vi "Initialize.vi"(8 "error in (no error)":errorcluster, 11 "NI Galvo in":refnum<class "NI Galvo.lvclass">) -> (0 "error out":errorcluster, 3 "NI Galvo out":refnum<class "NI Galvo.lvclass">)   [LabVIEW 2014, in "NI Galvo.lvclass"]
uses:
  NI Galvo.lvclass
  NI Galvo.lvclass/NI Galvo.ctl
  <vilib>/DAQmx/create/channels.llb/DAQmx Create Channel (AO-Voltage-Basic).vi
  <vilib>/DAQmx/configure/timing.llb/DAQmx Timing (Sample Clock).vi
  <vilib>/DAQmx/write.llb/DAQmx Write (Analog 2D DBL NChan NSamp).vi
  Galvo.lvclass
  <resource>/objmgr/daqmx.rc
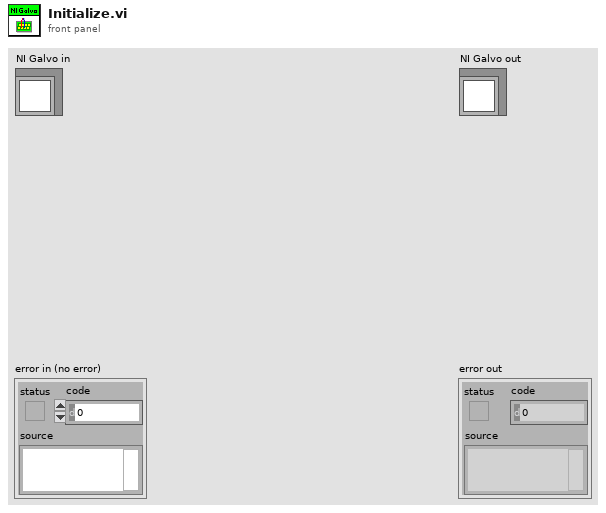
[diagram p1: front panel]
types:
  T1 = typedef "DAQ Class.lvclass/DAQ Parameters.ctl" = cluster{"Points Per A-Scan":u32, "A-Scans Per B-Scan":u32, "Number of B-Scans":u32, "A-Scans Per Transfer":u32, "Trigger Voltage":sgl, "Trigger Source":T2, "Trigger Slope":T3, "Channel":T4, "Clock":T5, "Bits per Sample":dbl, "Range":dbl}
  T2 = typedef "DAQ Class.lvclass/Trigger Source.ctl" = enum16{"External", "Channel A", "Channel B"}
  T3 = typedef "DAQ Class.lvclass/Trigger Slope.ctl" = enum16{"Rising", "Falling"}
  T4 = typedef "OCT DAQ Channel Data Type.ctl" = enum16{"Channel 1", "Channel 2", "Channel 1 and 2"}
  T5 = typedef "DAQ Class.lvclass/Clock Control.ctl" = enum16{"Internal Clock", "External Clock"}
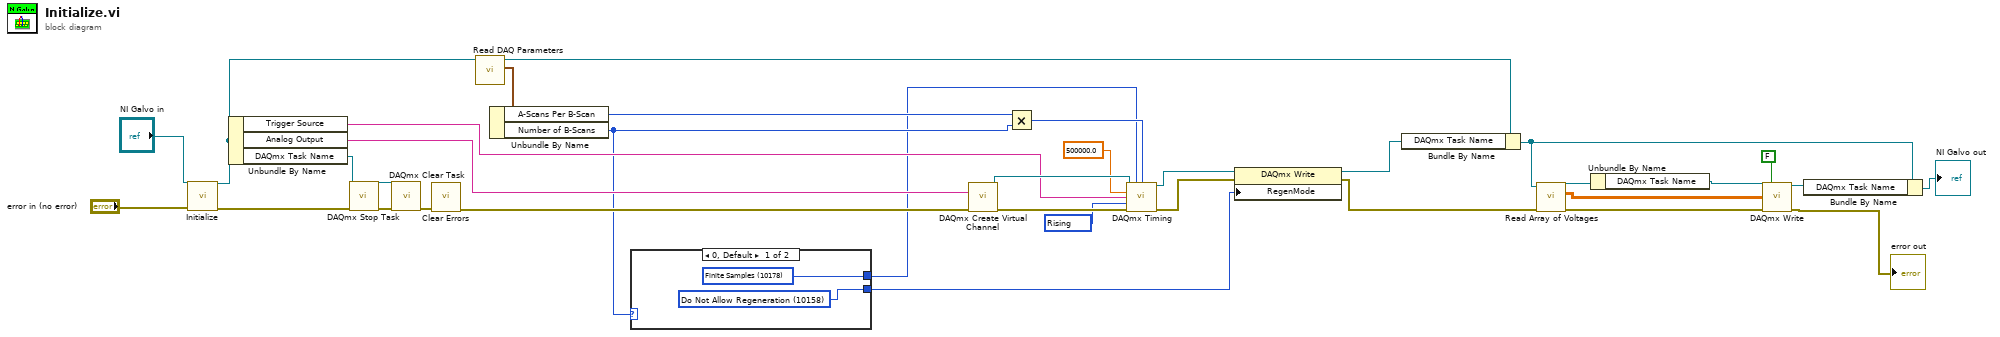
[diagram p0: block diagram]
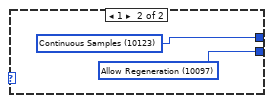
[diagram p2: hidden frame]
diagram:
  w27 = 10280 items=["Rising"=10280, "Falling"=10171] ("active edge")
  n1 = call-parent "Initialize.vi"("error in (no error)"="error in (no error)", "Galvo in"="NI Galvo in") -> ("error out"=w15:errorcluster, "Galvo out"=w17:refnum<class "NI Galvo.lvclass">)  [unwired: 8 in]
  n2 = Unbundle By Name(w17) -> ("Trigger Source"=w31:tag, "Analog Output"=w33:tag, "DAQmx Task Name"=w16:refnum<k21>)
  n3 = call <vilib>:"DAQmx Stop Task.vi"("task/channels in"=w16, "error in"=w15) -> ("task out"=w14:refnum<k21>, "error out"=w13:errorcluster)  [unwired: 12 in]
  n4 = call <vilib>:"DAQmx Clear Task.vi"("task in"=w14, "error in"=w13) -> ("error out"=w12:errorcluster)  [unwired: 13 in]
  n5 = call <vilib>:"Clear Errors.vi"("error in (no error)"=w12) -> ("error out"=w11:errorcluster)  [unwired: 5 in, 1 out]
  n6 = call-dynamic "Read DAQ Parameters.vi"("Galvo in"=w17) -> ("DAQ Parameters"=w19:T1, "Galvo out"=w20:refnum<class "NI Galvo.lvclass">)  [unwired: 8 in, 1 out]
  n7 = Unbundle By Name(w19) -> ("A-Scans Per B-Scan"=w18:u32, "Number of B-Scans"=w10:u32)
  n8 = case shown="0, Default" w10 {
    tunnel: [w37 w39] -> w1
    tunnel: [w36 w38] -> w8
    frame 0, Default {
      w36 = 10178 items=["Finite Samples"=10178, "Continuous Samples"=10123, "Hardware Timed Single Point"=12522] ("sample mode")
      w37 = 10158 items=["Allow Regeneration"=10097, "Do Not Allow Regeneration"=10158] ("RegenMode")
    }
    frame 1 {
      w38 = 10123 items=["Finite Samples"=10178, "Continuous Samples"=10123, "Hardware Timed Single Point"=12522] ("sample mode")
      w39 = 10097 items=["Allow Regeneration"=10097, "Do Not Allow Regeneration"=10158] ("RegenMode")
    }
  }
  n9 = call-poly <vilib>:"DAQmx Create Virtual Channel.vi"("physical channels"=w33, "error in"=w11) -> ("task out"=w32:refnum<k21>, "error out"=w30:errorcluster)  [unwired: 12 in]
  n10 = Multiply(x=w18, y=w10) -> (x*y=w28:u32)
  n11 = call-poly <vilib>:"DAQmx Timing.vi"("task/channels in"=w32, "sample mode"=w8, "samples per channel"=w28, "rate"=500000.0, "source"=w31, "active edge"=w27, "error in"=w30) -> ("task out"=w3:refnum<k21>, "error out"=w2:errorcluster)  [unwired: 7 in]
  n12 = property class="DAQmx Write"(reference=w3, error in=w2, "RegenMode"=w1) -> (reference out=w6:refnum<k21>, error out=w5:errorcluster)
  n13 = Bundle By Name(cluster=w20, "DAQmx Task Name"=w6) -> (w21:refnum<class "NI Galvo.lvclass">)
  n14 = call-dynamic "Read Array of Voltages.vi"("error in (no error)"=w5, "Galvo in"=w21) -> ("error out"=w22:errorcluster, "Array of Voltages"=w23:dbl[][], "Galvo out"=w25:refnum<class "NI Galvo.lvclass">)  [unwired: 7 in]
  n15 = Unbundle By Name(w25) -> ("DAQmx Task Name"=w24:refnum<k21>)
  n16 = call-poly <vilib>:"DAQmx Write.vi"("task/channels in"=w24, "auto start"=FALSE, "data"=w23, "error in"=w22) -> ("task out"=w7:refnum<k21>, "error out"=→"error out":errorcluster)  [unwired: 9 in, 1 out]
  n17 = Bundle By Name(cluster=w21, "DAQmx Task Name"=w7) -> (→"NI Galvo out":refnum<class "NI Galvo.lvclass">)
